vi "Brute Force Measurment SubVI.vi"(3 "Stop Program Brute Force":bool, 4 "Barcodes in":string[](array[string]), 5 "Channel # in":i32, 6 "Last Tube #":i32, 7 "error in (no error)":errorcluster, 9 "BoardHandle in":T1) -> (11 "Actual Voltage Level (V) 2":dbl format="%#_13g", 12 "Individual Tube Current (Nano Amps)":dbl[](array[numeric]), 13 "Failed Tubes":string[](array[string]), 18 "error out":errorcluster, 19 "BoardHandle out":T1)   [LabVIEW 2020]
panel:
  # "Pin in."
  # "Output pin positions"
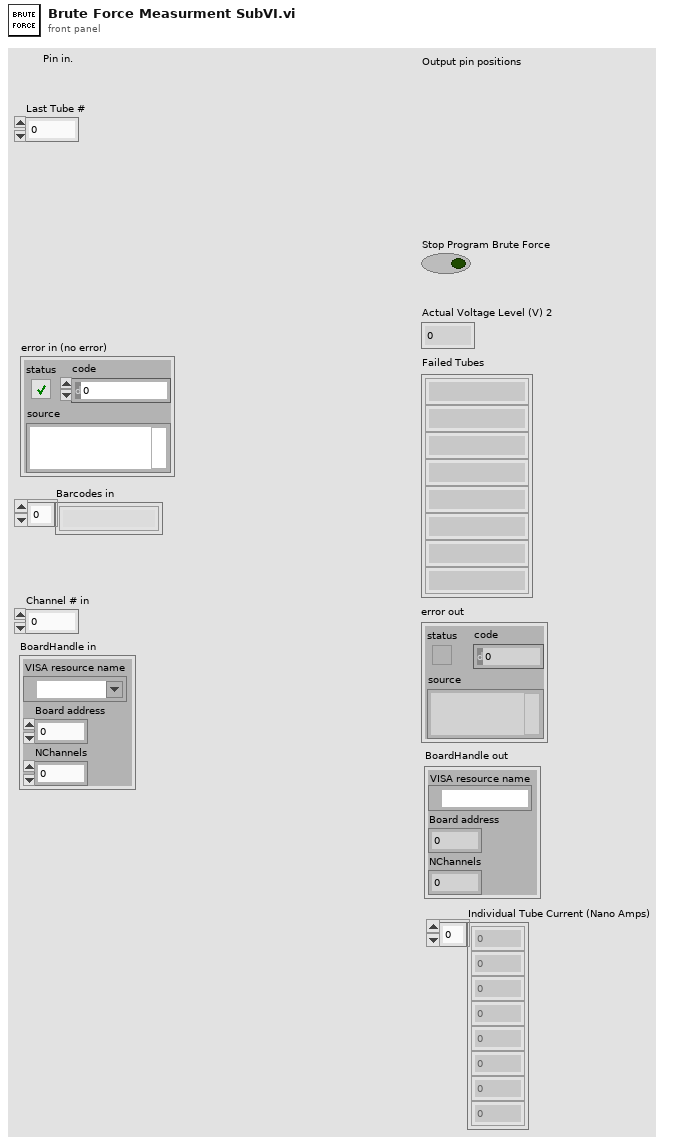
[diagram p1: front panel]
types:
  T1 = cluster{"VISA resource name":refnum<visa-resource-name>, "Board address":u8, "NChannels":u8}
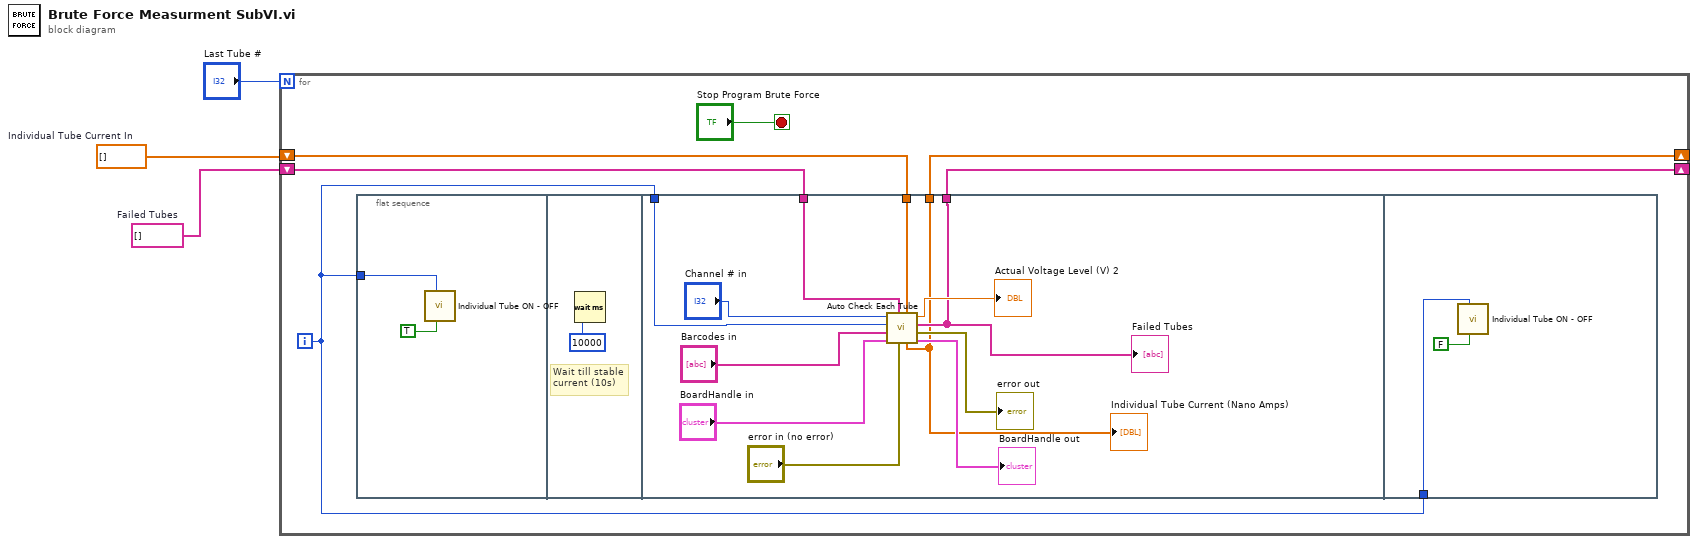
[diagram p0: block diagram]
diagram:
  w2 = dbl[] []  # Individual Tube Current In
  w3 = string[] []  # Failed Tubes
  n1 = for {
    N: "Last Tube #" -> [_]
    shift-right: [w7] -> _
    shift-left: w3 -> [w8]
    shift-right: [w5] -> _
    shift-left: w2 -> [w6]
    i -> [w9]
    stop <- "Stop Program Brute Force" stop-if-true
    n2 = flat-sequence {
      tunnel: w9 -> [w11]
      tunnel: w9 -> [w17]
      tunnel: w8 -> [w16]
      tunnel: [w15] -> w7
      tunnel: w6 -> [w14]
      tunnel: [w13] -> w5
      tunnel: w9 -> [w26]
      frame #0 {
        n3 = call "Individual Tube ON - OFF.vi"("Single Tube ON/OFF"=TRUE, "Tube #"=w11) -> ()  [unwired: 10 in]
      }
      frame #1 {
        # "Wait till stable\ncurrent (10s)"
        n4 = Wait (ms)(milliseconds to wait=u32 10000) -> ()  [unwired: 1 out]
      }
      frame #2 {
        n5 = call "Auto Check Each Tube.vi"("Individual Tube Current In"=w14, "error in (no error)"="error in (no error)", "Failed Tubes In"=w16, "BoardHandle in"="BoardHandle in", "Barcodes in"="Barcodes in", "Tube #"=w17, "Channel # in"="Channel # in") -> ("BoardHandle out"=→"BoardHandle out":T1, "error out"=→"error out":errorcluster, "Failed Tubes"=w15:string[], "Actual Voltage Level (V) 2"=→"Actual Voltage Level (V) 2":dbl, "Individual Tube Current (Nano Amps)"=w13:dbl[])
        "Failed Tubes" <- w15
        "Individual Tube Current (Nano Amps)" <- w13
      }
      frame #3 {
        n6 = call "Individual Tube ON - OFF.vi"("Single Tube ON/OFF"=FALSE, "Tube #"=w26) -> ()  [unwired: 10 in]
      }
    }
  }
